vi "Assert Less Or Equal_Variant.vi"(4 "Execution time (s)":dbl=-1.0, 5 "Assert Only? (F)":bool, 6 "error code (1)":i32=1, 7 "Label":string, 8 "error in (no error)":errorcluster, 10 "Y":variant, 11 "X":variant) -> (0 "error out":errorcluster)   [LabVIEW 2013, in "Caraya.lvlib" / "Assert.lvclass"]
doc: "Generates an error if the input condition is not met.\n\n--\nCopyright © 2015 JKI All rights reserved.\n\nAuthor: Tomi Maila <tomi.maila@jki.net>\n\nThis library is provided \"AS IS\" ,WITHOUT WARRANTIES OR\nCONDITIONS OF ANY KIND, either express or implied.\n\nJKI -- jki.net"
uses:
  Assert.lvclass
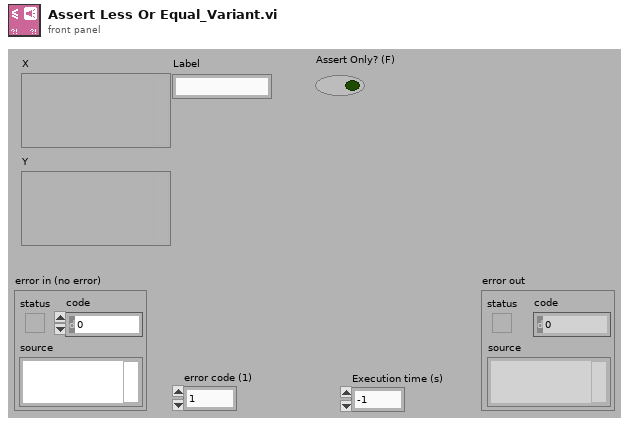
[diagram p1: front panel]
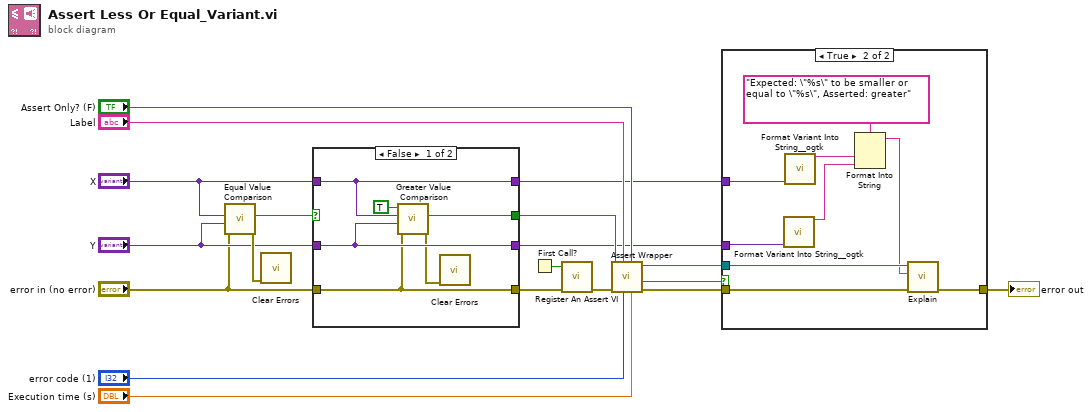
[diagram p0: block diagram]
diagram:
  n1 = call "Equal Value Comparison.vi"("error in (no error)"="error in (no error)", "Y"="Y", "X"="X") -> ("error out"=w10:errorcluster, "Equal Values?"=w11:bool)  [unwired: 6 in, 1 out]
  n2 = call <vilib>:"Clear Errors.vi"("error in (no error)"=w10) -> ()  [unwired: 6 in, 1 out]
  n3 = case shown="False" w11 {
    selector: w11 -> [_ w28]
    tunnel: "X" -> [w25 w29]
    tunnel: [w25 w29] -> w8
    tunnel: [w23 w28] -> w9
    tunnel: "Y" -> [w24 w27]
    tunnel: [w24 w27] -> w5
    tunnel: "error in (no error)" -> [w22 w26]
    tunnel: [w22 w26] -> w2
    frame False {
      n4 = call "Greater Value Comparison.vi"("error in (no error)"=w22, "Y"=w24, "X"=w25, "Less Than? (F)"=TRUE) -> ("error out"=w21:errorcluster, "Asserted?"=w23:bool)  [unwired: 5 in, 1 out]
      n5 = call <vilib>:"Clear Errors.vi"("error in (no error)"=w21) -> ()  [unwired: 6 in, 1 out]
    }
    frame True {
    }
  }
  n6 = First Call?() -> (First Call?: T/F=w3:bool)
  n7 = call "Register An Assert VI.vi"("error in (no error)"=w2, "first call?"=w3) -> ("error out"=w1:errorcluster)  [unwired: 9 in]
  n8 = call "Assert Wrapper.vi"("Execution time (s)"="Execution time (s)", "Assert Only? (F)"="Assert Only? (F)", "error code (1)"="error code (1)", "Label"="Label", "error in (no error)"=w1, "Assert?"=w9) -> ("error out"=w15:errorcluster, "Verbose"=w13:bool, "Assert out"=w12:refnum<class "Assert.lvclass">)  [unwired: 3 in]
  n9 = case shown="True" w13 {
    tunnel: [w30 w39] -> w14
    tunnel: w12 -> [_ w38]
    tunnel: w15 -> [w30 w37]
    tunnel: w8 -> [_ w35]
    tunnel: w5 -> [_ w34]
    frame False {
    }
    frame True {
      n10 = call <userlib>:"Format Variant Into String__ogtk.vi"("Variant"=w34) -> ("Output String"=w31:string)  [unwired: 13 in, 1 out]
      n11 = call <userlib>:"Format Variant Into String__ogtk.vi"("Variant"=w35) -> ("Output String"=w32:string)  [unwired: 13 in, 1 out]
      n12 = Format Into String(format string="Expected: \"%s\" to be smaller or equal to \"%s\", Asserted: greater" ("t"), w32, w31) -> (resulting string=w36:string)  [unwired: 2 in, 1 out]
      n13 = call "Explain.vi"("error in (no error)"=w37, "Verbose Explanation"=w36, "Assert in"=w38) -> ("error out"=w39:errorcluster)  [unwired: 7 in, 1 out]
    }
  }
  "error out" <- w14
